vi "save user config file.vi"(11 "config parameters":T13 {"messageHandler"."params"."controlChannels"."ballControl" items=["Module6/output0", "Module6/output1", "Module6/output2", "Module6/output3", "Not-Used"]; "messageHandler"."params"."controlChannels"."butterflyControl" items=["Module6/output0", "Module6/output1", "Module6/output2", "Module6/output3", "Not-Used"]; "messageHandler"."params"."controlChannels"."speedControl" items=["Module6/output0", "Module6/output1", "Module6/output2", "Module6/output3", "Not-Used"]}) -> ()   [LabVIEW 2018]
uses:
  type defs/message handler data.ctl
  customVI/liveData/state.ctl
  type defs/comms loop data.ctl
  ICL-LabVIEW_General/Incident logger/Incident logger.lvclass
  <vilib>/Modbus/master/Modbus Master.lvclass
  type defs/data stream data.ctl
  type defs/data processor data.ctl
  type defs/channelLimitControl.ctl
  type defs/limitActions.ctl
  type defs/file IO data.ctl
  type defs/channelControl.ctl
  RT/Type Defs/channelScalingTypes.ctl
  RT/Type Defs/scalingMethods.ctl
  ICL-LabVIEW_General/data channels/parent class/Data Channel.lvclass
  type defs/UI loop data.ctl
  type defs/error messages data.ctl
  <vilib>/Utility/config.llb/Write Key (String).vi
  <vilib>/Utility/config.llb/Write Key (Path).vi
  <vilib>/Utility/config.llb/Write Key (U32).vi
  <vilib>/Utility/config.llb/NI_LVConfig.lvlib
panel:
  out "error out 2":errorcluster
  out "error out":errorcluster
  out "unwritten keys":string[](array[string])
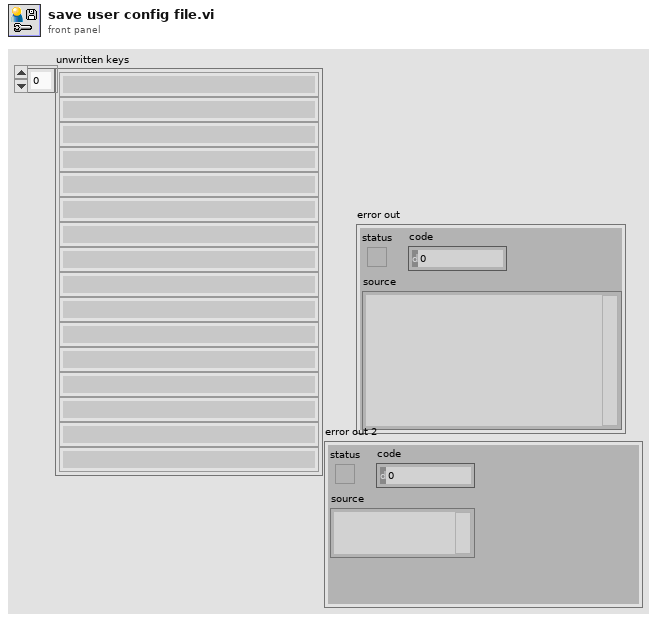
[diagram p1: front panel]
types:
  T1 = typedef "message handler data.ctl" = cluster{"params":cluster{"configFileID":u32, "configFilePath":path, "channelConfigFilePath":path, "incidentLogfile":path, "controlChannels":cluster{"ballControl":u16, "butterflyControl":u16, "speedControl":u16}, "pulsatorVIPath":path, "customVIPath":path, "HowdenAir":cluster{"vent Howden":bool, "Howden%":dbl}}, "vars":cluster{"commsStatus":bool[], "controlIndex":cluster{"ballControl":u16, "butterflyControl":u16, "speedControl":u16}, "customVIRef":refnum<vi>, "Interlocks":cluster{"gearboxOil":bool, "bearingOil":bool, "gearboxAir":bool}, "motorRunning":bool, "liveDataQ":refnum<queue>[]}}
  T2 = typedef "comms loop data.ctl" = cluster{"params":cluster{"commandStream":cluster{"reader name":string, "writer name":string, "stream buffer size":i32}, "errorStream":cluster{"reader name":string, "writer name":string, "stream buffer size":i32}, "RT IP address":string, "pulserControllerIP":string}, "vars":cluster{"commandStream":refnum<k21>, "Incident logger":refnum<class "Incident logger.lvclass">, "check error scheduled message":u32, "errorStream":refnum<k21>, "watchdogScheduleID":u32, "pulsator":cluster{"pulser connection":refnum<class "Modbus Master.lvclass">, "pulserConnected":bool, "pulsatorScheduleID":u32, "pulserRunning":bool, "pulsatorRetries":u8}}}
  T3 = typedef "data stream data.ctl" = cluster{"params":cluster{"Stream":cluster{"reader name":string, "RT IP address":string, "writer name":string, "stream buffer size":i32}}, "vars":cluster{"data stream":refnum<k21>}}
  T4 = typedef "data processor data.ctl" = cluster{"params":cluster{"controlFeedback":cluster{"butterflyValue":u16, "ballValue":u16, "massflow":u16, "pressureRatio":u16, "compSpeed":u16}, "DAQrate":enum16{"50 kHz", "25 kHz", "16.6 kHz", "12.5 kHz", "10 kHz", "8.33 kHz", "7.14 kHz", "6.25 kHz", "5.55 kHz", "5 kHz"}, "safetyChannels":cluster{"oilP":u16, "airP":u16, "water":u16, "channelLimit":T5[]}, "channelConfigPath":path}, "vars":cluster{"controlFeedback":cluster{"butterflyValue":u16, "ballValue":u16, "massflow":u16, "pressureRatio":u16, "compSpeed":u16}, "activeChannelNames":string[], "activeChannelUnits":string[], "offset trigger":bool, "offsets":dbl[], "activeChannelLimitIndex":u16[], "liveData":bool}}
  T5 = typedef "channelLimitControl.ctl" = cluster{"channelID":u16, "Enabled":bool, "warnValue":dbl, "limitValue":dbl, "Invert":bool, "limitAction":T6}
  T6 = typedef "limitActions.ctl" = enum16{"stop", "shutdown", "ignore"}
  T7 = typedef "file IO data.ctl" = cluster{"params":cluster{"startFolder":path, "channelConfigPath":path}, "vars":cluster{"channelConfig ":T8[], "writing":cluster{"streaming":bool, "fixedLength":bool, "pointCount":u32, "timeZero":dbl, "pointsWritten":u32, "dataRate":u16}, "channelCount":u16, "fileTarget":cluster{"Save folder":path, "Target filename":string, "file ref":refnum<file>, "pulsatorSpeed":string, "motorSpeed":string, "valvePosition":string, "torqueFilter":bool, "pulsatorRunning":bool, "motorRunning":bool}, "channels":refnum<class "Data Channel.lvclass">[]}}
  T8 = typedef "channelControl.ctl" = cluster{"index":u16, "active":bool, "channelType":T9, "module":u16, "terminal":u16, "channelName":string, "scalingMethod":T10, "scalingParameters":dbl[], "scaledUnits":string, "tempOffset":dbl}
  T9 = typedef "channelScalingTypes.ctl" = enum16{"calculation", "measurement", "scanivalve", "output", "digital"}
  T10 = typedef "scalingMethods.ctl" = enum16{"none", "linear", "thermocouple", "polynomial", "encoder", "RTD"}
  T11 = typedef "UI loop data.ctl" = cluster{"params":cluster{"channelConfigPath":path, "version":string}, "vars":cluster{"tempOffsets":dbl[], "encoderFallingEdge":bool, "controlRefs":cluster{"mainVI":refnum<vi>, "menu":refnum<k9>, "motorStart":refnum<vi>, "butterfly":refnum<vi>, "ball":refnum<vi>, "speed":refnum<vi>, "logLimit":refnum<vi>, "pointLimit":refnum<vi>, "logData":refnum<vi>}}}
  T12 = typedef "error messages data.ctl" = cluster{"params":cluster{"eg":bool}, "vars":cluster{"eg":bool}}
  T13 = cluster{"messageHandler":T1, "comms":T2, "dataStream":T3, "dataProcessor":T4, "fileIO":T7, "userInterface":T11, "errors":T12}
  T14 = typedef "NI_LVConfig.lvlib/Config Data RefNum.ctl" = refnum<k1>
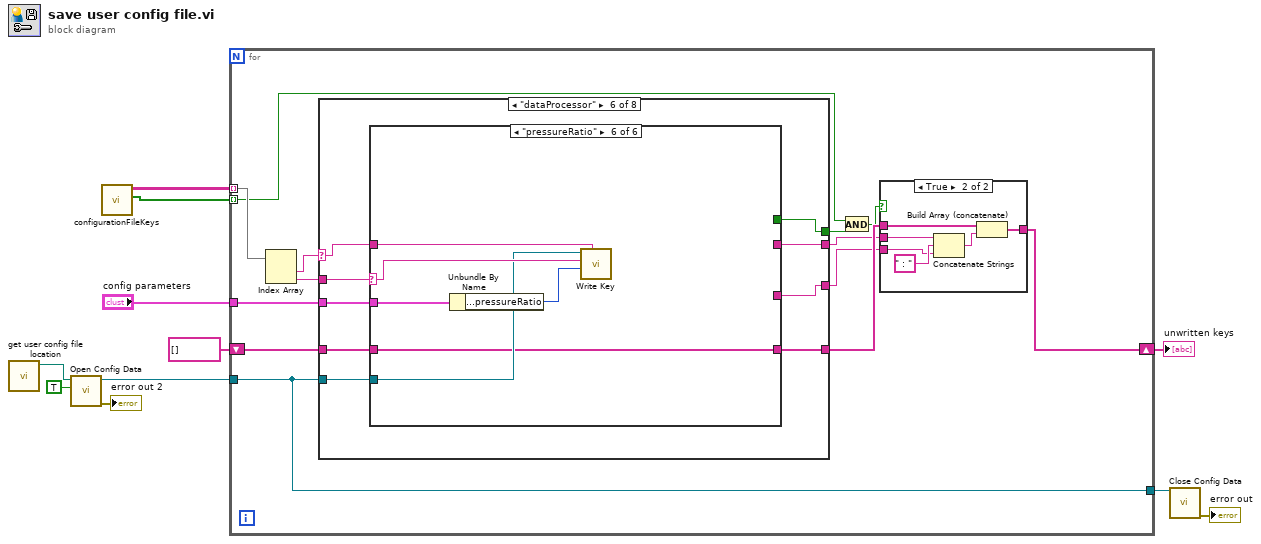
[diagram p0: block diagram]
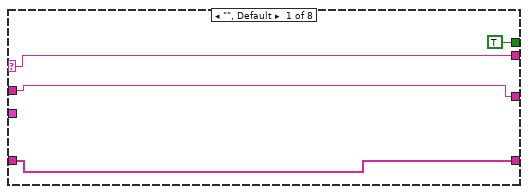
[diagram p3: hidden frame]
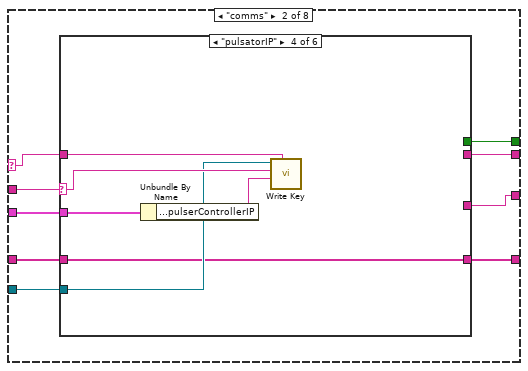
[diagram p4: hidden frame]
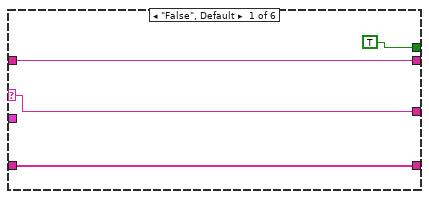
[diagram p5: hidden frame]
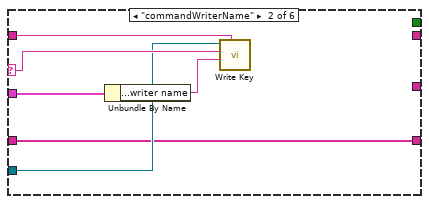
[diagram p6: hidden frame]
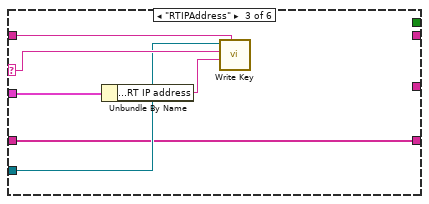
[diagram p7: hidden frame]
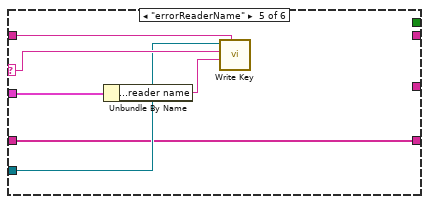
[diagram p8: hidden frame]
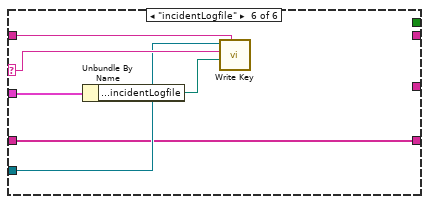
[diagram p9: hidden frame]
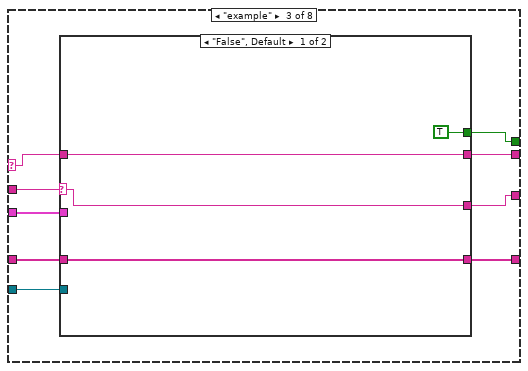
[diagram p10: hidden frame]
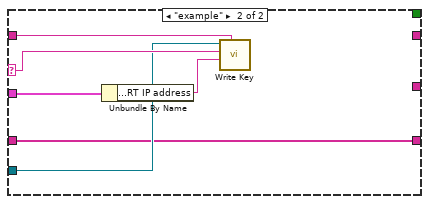
[diagram p11: hidden frame]
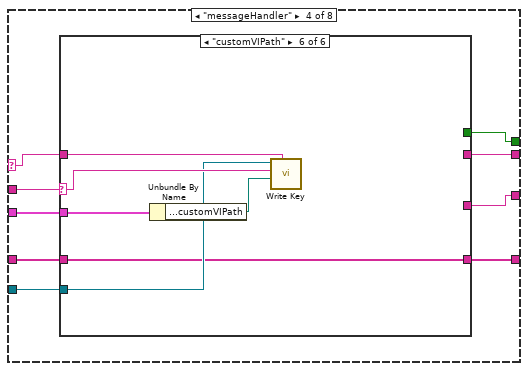
[diagram p12: hidden frame]
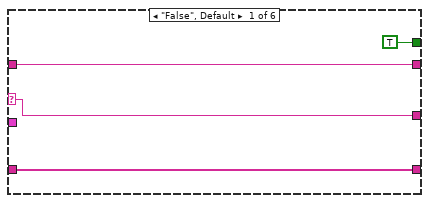
[diagram p13: hidden frame]
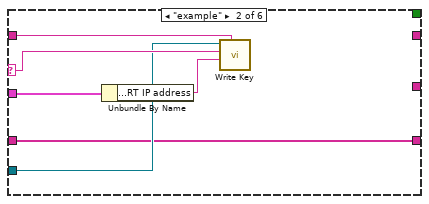
[diagram p14: hidden frame]
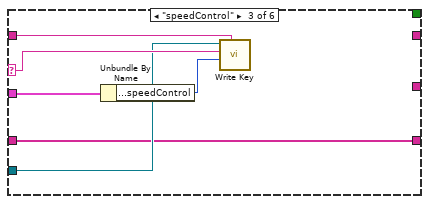
[diagram p15: hidden frame]
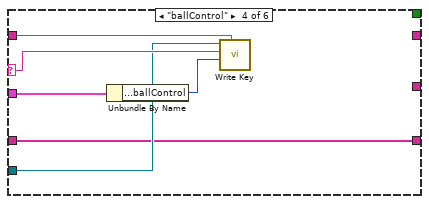
[diagram p16: hidden frame]
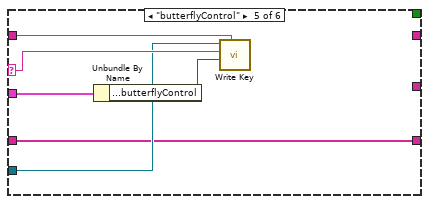
[diagram p17: hidden frame]
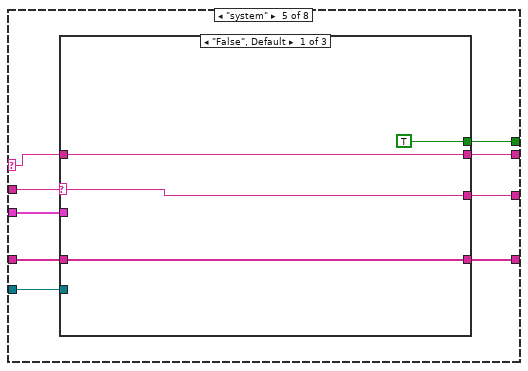
[diagram p18: hidden frame]
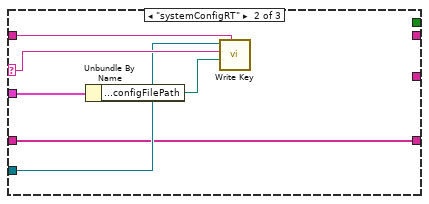
[diagram p19: hidden frame]
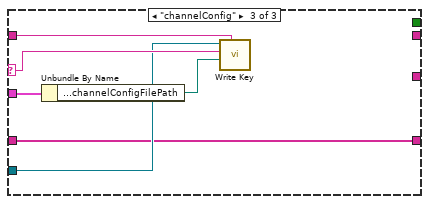
[diagram p20: hidden frame]
diagram:
  n1 = call "get user config file location.vi"() -> ("userConfigPath"=w9:path)  [unwired: 11 in]
  n2 = call <vilib>:"Open Config Data.vi"("create file if necessary (T)"=TRUE, "configuration file path"=w9) -> ("error out"=→"error out 2":errorcluster, "refnum"=w8:T14)  [unwired: 7 in, 1 out]
  n3 = call "configurationFileKeys.vi"() -> ("write user key?"=w3:bool[], "userConfigKeys"=w10:string[][])  [unwired: 9 in, 1 out]
  n4 = for {
    tunnel: "config parameters" -> [w20]
    tunnel: w10 -> [w24] mode=indexing
    tunnel: w8 -> [w21]
    tunnel: [w21] -> w7
    shift-right: [w17] -> w4
    shift-left: string[] [] -> [w19]
    tunnel: w3 -> [w15] mode=indexing
    n5 = Index Array(array=w24) -> (element #1=w23:string, element #2=w22:string)  [unwired: 2 in]
    n6 = case shown="\"dataProcessor\"" w23 {
      selector: w23 -> [w35 w41 w84 w103 w146 w171 w214 w233]
      tunnel: w22 -> [w34 w44 w87 w106 w149 w174 w217 w236]
      tunnel: w21 -> [_ w43 w86 w105 w148 w173 w216 w235]
      tunnel: w20 -> [_ w42 w85 w104 w147 w172 w215 w234]
      tunnel: [w33 w40 w83 w102 w145 w170 w213 w232] -> w18
      tunnel: w19 -> [w33 w39 w82 w101 w144 w169 w212 w231]
      tunnel: [TRUE w36 w79 w98 w143 w166 w209 w228] -> w16
      tunnel: [w35 w38 w81 w100 w142 w168 w211 w230] -> w13
      tunnel: [w34 w37 w80 w99 w141 w167 w210 w229] -> w12
      frame "", Default {
      }
      frame "comms" {
        n7 = case shown="\"pulsatorIP\"" w44 {
          selector: w44 -> [w46 w53 w59 w65 w71 w77]
          tunnel: w43 -> [_ w52 w58 w64 w70 w76]
          tunnel: w42 -> [_ w51 w57 w63 w69 w75]
          tunnel: w41 -> [w47 w54 w60 w66 w72 w78]
          tunnel: [w48 w49 w55 w61 w67 w73] -> w40
          tunnel: w39 -> [w48 w49 w55 w61 w67 w73]
          tunnel: [w47 _ _ _ _ _] -> w38
          tunnel: [w46 _ _ _ _ _] -> w37
          tunnel: [TRUE _ _ _ _ _] -> w36
          frame "False", Default {
          }
          frame "commandWriterName" {
            n8 = Unbundle By Name(w51) -> ("comms.params.commandStream.writer name"=w50:string)
            n9 = call-poly <vilib>:"Write Key.vi"("section"=w54, "value"=w50, "key"=w53, "refnum"=w52) -> ()  [unwired: 5 in, 3 out]
          }
          frame "RTIPAddress" {
            n10 = Unbundle By Name(w57) -> ("comms.params.RT IP address"=w56:string)
            n11 = call-poly <vilib>:"Write Key.vi"("section"=w60, "value"=w56, "key"=w59, "refnum"=w58) -> ()  [unwired: 5 in, 3 out]
          }
          frame "pulsatorIP" {
            n12 = Unbundle By Name(w63) -> ("comms.params.pulserControllerIP"=w62:string)
            n13 = call-poly <vilib>:"Write Key.vi"("section"=w66, "value"=w62, "key"=w65, "refnum"=w64) -> ()  [unwired: 5 in, 3 out]
          }
          frame "errorReaderName" {
            n14 = Unbundle By Name(w69) -> ("comms.params.errorStream.reader name"=w68:string)
            n15 = call-poly <vilib>:"Write Key.vi"("section"=w72, "value"=w68, "key"=w71, "refnum"=w70) -> ()  [unwired: 5 in, 3 out]
          }
          frame "incidentLogfile" {
            n16 = Unbundle By Name(w75) -> ("messageHandler.params.incidentLogfile"=w74:path)
            n17 = call-poly <vilib>:"Write Key.vi"("section"=w78, "value"=w74, "key"=w77, "refnum"=w76) -> ()  [unwired: 5 in, 3 out]
          }
        }
      }
      frame "example" {
        n18 = case shown="\"False\", Default" w87 {
          selector: w87 -> [w89 w96]
          tunnel: w86 -> [_ w95]
          tunnel: w85 -> [_ w94]
          tunnel: w84 -> [w90 w97]
          tunnel: [w91 w92] -> w83
          tunnel: w82 -> [w91 w92]
          tunnel: [w90 _] -> w81
          tunnel: [w89 _] -> w80
          tunnel: [TRUE _] -> w79
          frame "False", Default {
          }
          frame "example" {
            n19 = Unbundle By Name(w94) -> ("comms.params.RT IP address"=w93:string)
            n20 = call-poly <vilib>:"Write Key.vi"("section"=w97, "value"=w93, "key"=w96, "refnum"=w95) -> ()  [unwired: 5 in, 3 out]
          }
        }
      }
      frame "messageHandler" {
        n21 = case shown="\"customVIPath\"" w106 {
          selector: w106 -> [w108 w115 w121 w127 w133 w139]
          tunnel: w105 -> [_ w114 w120 w126 w132 w138]
          tunnel: w104 -> [_ w113 w119 w125 w131 w137]
          tunnel: w103 -> [w109 w116 w122 w128 w134 w140]
          tunnel: [w110 w111 w117 w123 w129 w135] -> w102
          tunnel: w101 -> [w110 w111 w117 w123 w129 w135]
          tunnel: [w109 _ _ _ _ _] -> w100
          tunnel: [w108 _ _ _ _ _] -> w99
          tunnel: [TRUE _ _ _ _ _] -> w98
          frame "False", Default {
          }
          frame "example" {
            n22 = Unbundle By Name(w113) -> ("comms.params.RT IP address"=w112:string)
            n23 = call-poly <vilib>:"Write Key.vi"("section"=w116, "value"=w112, "key"=w115, "refnum"=w114) -> ()  [unwired: 5 in, 3 out]
          }
          frame "speedControl" {
            n24 = Unbundle By Name(w119) -> ("messageHandler.params.controlChannels.speedControl"=w118:u16)
            n25 = call-poly <vilib>:"Write Key.vi"("section"=w122, "value"=w118, "key"=w121, "refnum"=w120) -> ()  [unwired: 5 in, 3 out]
          }
          frame "ballControl" {
            n26 = Unbundle By Name(w125) -> ("messageHandler.params.controlChannels.ballControl"=w124:u16)
            n27 = call-poly <vilib>:"Write Key.vi"("section"=w128, "value"=w124, "key"=w127, "refnum"=w126) -> ()  [unwired: 5 in, 3 out]
          }
          frame "butterflyControl" {
            n28 = Unbundle By Name(w131) -> ("messageHandler.params.controlChannels.butterflyControl"=w130:u16)
            n29 = call-poly <vilib>:"Write Key.vi"("section"=w134, "value"=w130, "key"=w133, "refnum"=w132) -> ()  [unwired: 5 in, 3 out]
          }
          frame "customVIPath" {
            n30 = Unbundle By Name(w137) -> ("messageHandler.params.customVIPath"=w136:path)
            n31 = call-poly <vilib>:"Write Key.vi"("section"=w140, "value"=w136, "key"=w139, "refnum"=w138) -> ()  [unwired: 5 in, 3 out]
          }
        }
      }
      frame "system" {
        n32 = case shown="\"False\", Default" w149 {
          selector: w149 -> [w150 w158 w164]
          tunnel: w148 -> [_ w157 w163]
          tunnel: w147 -> [_ w156 w162]
          tunnel: w146 -> [w151 w159 w165]
          tunnel: [w153 w154 w160] -> w145
          tunnel: w144 -> [w153 w154 w160]
          tunnel: [TRUE _ _] -> w143
          tunnel: [w151 _ _] -> w142
          tunnel: [w150 _ _] -> w141
          frame "False", Default {
          }
          frame "systemConfigRT" {
            n33 = Unbundle By Name(w156) -> ("messageHandler.params.configFilePath"=w155:path)
            n34 = call-poly <vilib>:"Write Key.vi"("section"=w159, "value"=w155, "key"=w158, "refnum"=w157) -> ()  [unwired: 5 in, 3 out]
          }
          frame "channelConfig" {
            n35 = Unbundle By Name(w162) -> ("messageHandler.params.channelConfigFilePath"=w161:path)
            n36 = call-poly <vilib>:"Write Key.vi"("section"=w165, "value"=w161, "key"=w164, "refnum"=w163) -> ()  [unwired: 5 in, 3 out]
          }
        }
      }
      frame "dataProcessor" {
        n37 = case shown="\"pressureRatio\"" w174 {
          selector: w174 -> [w176 w183 w189 w195 w201 w207]
          tunnel: w173 -> [_ w182 w188 w194 w200 w206]
          tunnel: w172 -> [_ w181 w187 w193 w199 w205]
          tunnel: w171 -> [w177 w184 w190 w196 w202 w208]
          tunnel: [w178 w179 w185 w191 w197 w204] -> w170
          tunnel: w169 -> [w178 w179 w185 w191 w197 w204]
          tunnel: [w177 _ _ _ _ _] -> w168
          tunnel: [w176 _ _ _ _ _] -> w167
          tunnel: [TRUE _ _ _ _ _] -> w166
          frame "False", Default {
          }
          frame "speedChannel" {
            n38 = Unbundle By Name(w181) -> ("dataProcessor.params.controlFeedback.compSpeed"=w180:u16)
            n39 = call-poly <vilib>:"Write Key.vi"("section"=w184, "value"=w180, "key"=w183, "refnum"=w182) -> ()  [unwired: 5 in, 3 out]
          }
          frame "butterflyChannel" {
            n40 = Unbundle By Name(w187) -> ("dataProcessor.params.controlFeedback.butterflyValue"=w186:u16)
            n41 = call-poly <vilib>:"Write Key.vi"("section"=w190, "value"=w186, "key"=w189, "refnum"=w188) -> ()  [unwired: 5 in, 3 out]
          }
          frame "ballChannel" {
            n42 = Unbundle By Name(w193) -> ("dataProcessor.params.controlFeedback.ballValue"=w192:u16)
            n43 = call-poly <vilib>:"Write Key.vi"("section"=w196, "value"=w192, "key"=w195, "refnum"=w194) -> ()  [unwired: 5 in, 3 out]
          }
          frame "massflow" {
            n44 = Unbundle By Name(w199) -> ("dataProcessor.params.controlFeedback.massflow"=w198:u16)
            n45 = call-poly <vilib>:"Write Key.vi"("section"=w202, "value"=w198, "key"=w201, "refnum"=w200) -> ()  [unwired: 5 in, 3 out]
          }
          frame "pressureRatio" {
            n46 = Unbundle By Name(w205) -> ("dataProcessor.params.controlFeedback.pressureRatio"=w203:u16)
            n47 = call-poly <vilib>:"Write Key.vi"("section"=w208, "value"=w203, "key"=w207, "refnum"=w206) -> ()  [unwired: 5 in, 3 out]
          }
        }
      }
      frame "fileIO" {
        n48 = case shown="\"False\", Default" w217 {
          selector: w217 -> [w219 w226]
          tunnel: w216 -> [_ w225]
          tunnel: w215 -> [_ w224]
          tunnel: w214 -> [w220 w227]
          tunnel: [w221 w222] -> w213
          tunnel: w212 -> [w221 w222]
          tunnel: [w220 _] -> w211
          tunnel: [w219 _] -> w210
          tunnel: [TRUE _] -> w209
          frame "False", Default {
          }
          frame "startFolder" {
            n49 = Unbundle By Name(w224) -> ("fileIO.params.startFolder"=w223:path)
            n50 = call-poly <vilib>:"Write Key.vi"("section"=w227, "value"=w223, "key"=w226, "refnum"=w225) -> ()  [unwired: 5 in, 3 out]
          }
        }
      }
      frame "dataStream" {
        n51 = case shown="\"False\", Default" w236 {
          selector: w236 -> [w238 w245]
          tunnel: w235 -> [_ w244]
          tunnel: w234 -> [_ w243]
          tunnel: w233 -> [w239 w246]
          tunnel: [w240 w241] -> w232
          tunnel: w231 -> [w240 w241]
          tunnel: [w239 _] -> w230
          tunnel: [w238 _] -> w229
          tunnel: [TRUE _] -> w228
          frame "False", Default {
          }
          frame "dataReaderName" {
            n52 = Unbundle By Name(w243) -> ("dataStream.params.Stream.reader name"=w242:string)
            n53 = call-poly <vilib>:"Write Key.vi"("section"=w246, "value"=w242, "key"=w245, "refnum"=w244) -> ()  [unwired: 5 in, 3 out]
          }
        }
      }
    }
    n54 = And(x=w15, y=w16) -> (x .and. y?=w14:bool)
    n55 = case shown="True" w14 {
      tunnel: [w25 w28] -> w17
      tunnel: w18 -> [w25 w29]
      tunnel: w13 -> [_ w27]
      tunnel: w12 -> [_ w26]
      frame False {
      }
      frame True {
        n56 = Concatenate Strings(w27, " : " ("string"), w26) -> (w30:string)
        n57 = Build Array (concatenate)(w29, w30) -> (w28:string[])
      }
    }
  }
  "unwritten keys" <- w4
  n58 = call <vilib>:"Close Config Data.vi"("refnum"=w7) -> ("error out"=→"error out":errorcluster)  [unwired: 9 in, 1 out]
